vi "CPU.vi"(4 "Adr b":cluster{"a0":bool, "a1":bool}, 5 "Adr A":cluster{"a0":bool, "a1":bool}, 6 "c":bool, 7 "Func":T1, 8 "Cinp":bool, 9 "Reset":bool, 10 "Keyboard":T2, 11 "Minus":bool) -> (0 "flags":T4, 1 "dig1":T3, 2 "dig0":T3, 3 "sign":bool)   [LabVIEW 2013]
panel:
  # "Логические функции     \n  1001 - \"0\"\n  1010 - Adr A ^ Adr B\n  1011 - Adr A ^ ~Adr B\n  1100 - Adr A\n  1101 - ~Adr A ^ Adr B\n  1110 - Adr B\n  1111 - Adr A (+) Adr B\n10000 - Adr A \\/ Adr B\n10001 - ~Adr A ^ ~Adr B\n10010 - ~(Adr A (+) Adr B)\n10011 - ~Adr B\n10100 - Adr A \\/ ~Adr B\n10101 - ~Adr A\n10110 - ~Adr A \\/ Adr B\n10111 - ~Adr A \\/ ~Adr B\n11000 - \"1\""
  # "Арифметические функции\n    101 - Adr A + Adr B\n    110 - Acc + Adr B\n    111 - Adr A - Adr B\n  1000 - Acc - Adr B"
  # "0 - Очистка аккумулятора\n        1 - Ввод в память по адресу Adr A\n      10 - Запись аккумулятора в память по адресу Adr A\n      11 - Вывод из аккумулятора\n    100 - Вывод из памяти по адресу Adr B"
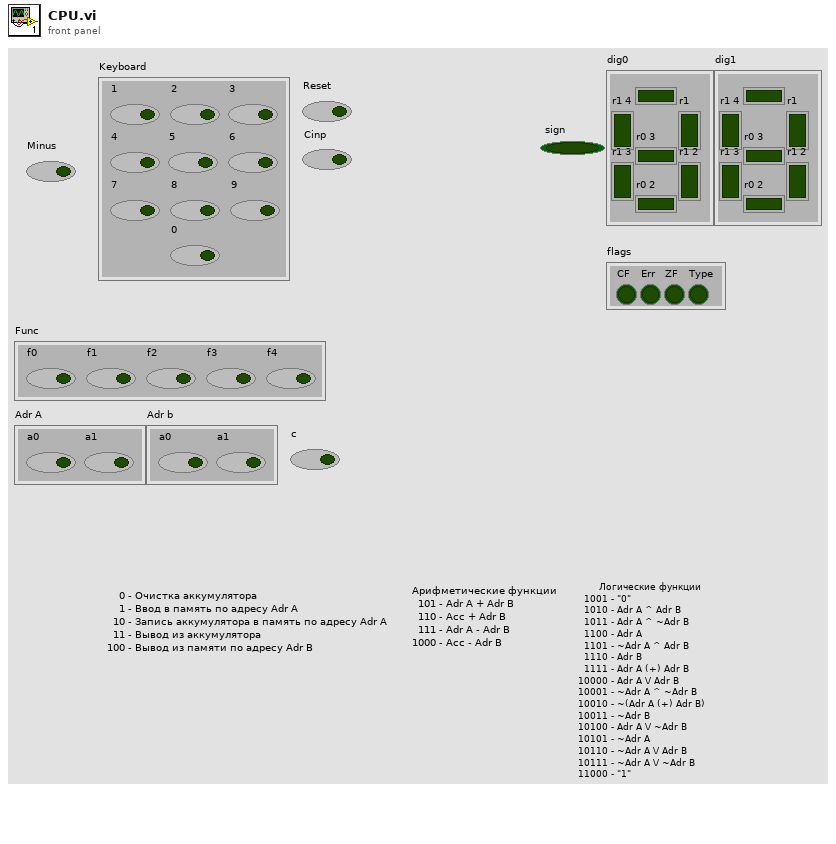
[diagram p1: front panel]
types:
  T1 = cluster{"f0":bool, "f1":bool, "f2":bool, "f3":bool, "f4":bool}
  T2 = cluster{"0":bool, "1":bool, "2":bool, "3":bool, "4":bool, "5":bool, "6":bool, "7":bool, "8":bool, "9":bool}
  T3 = cluster{"r0":bool, "r1":bool, "r1 2":bool, "r0 2":bool, "r1 3":bool, "r1 4":bool, "r0 3":bool}
  T4 = cluster{"CF":bool, "Err":bool, "ZF":bool, "Type":bool}
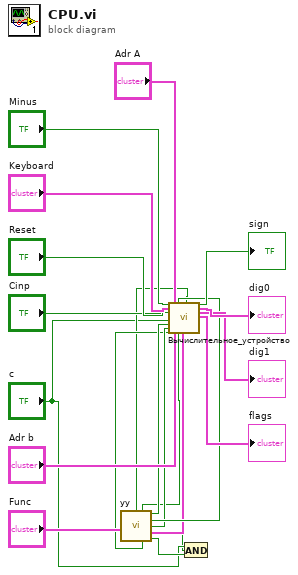
[diagram p0: block diagram]
diagram:
  n1 = call "УУ.vi"("Func"="Func") -> ("Read"=w4:bool, "Exec"=w5:bool, "SelInp"=w10:bool, "Wr"=w9:bool, "SelOp"=w8:bool, "ALU func"=w7:T1, "Cread"=w6:bool, "ClearAcc"=w3:bool)  [unwired: 7 in]
  n2 = And(x="c", y=w3) -> (x .and. y?=w1:bool)
  n3 = call "Вычислительное_устройство.vi"("Minus"="Minus", "Keyboard"="Keyboard", "Reset"="Reset", "Cinp"="Cinp", "c"="c", "selInp"=w10, "selOp"=w8, "Cread"=w6, "Adr A"="Adr A", "Adr b"="Adr b", "wr"=w9, "Exec"=w5, "ClearAcc"=w1, "Func"=w7, "read"=w4) -> ("sign"=→"sign":bool, "dig0"=→"dig0":T3, "dig1"=→"dig1":T3, "flags"=→"flags":T4)  [unwired: 9 in]
